vi "NanoValve Inject.vi"(8 "error in (no error)":errorcluster, 11 "VISA resource name":refnum<visa-resource-name>) -> (0 "error out":errorcluster)   [LabVIEW 2015]
uses:
  <vilib>/Instr/_visa.llb/VISA Configure Serial Port (Instr).vi
panel:
  out "return count":u32
  # "Inject Sample"
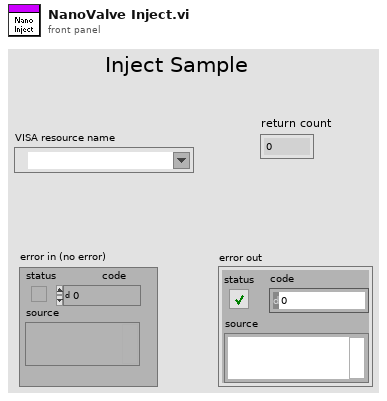
[diagram p1: front panel]
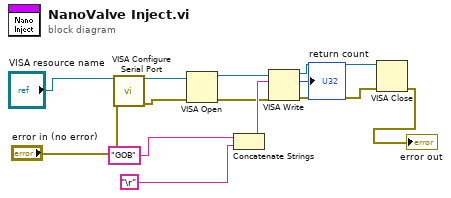
[diagram p0: block diagram]
diagram:
  n1 = call-poly "VISA Configure Serial Port"("VISA resource name"="VISA resource name", "error in (no error)"="error in (no error)") -> ("VISA resource name out"=w8:refnum<visa-resource-name>, "error out"=w7:errorcluster)  [unwired: 12 in]
  n2 = VISA Open(error in (no error)=w7, VISA resource name=w8) -> (VISA resource name=w10:refnum<visa-resource-name>, error out=w6:errorcluster)  [unwired: 3 in]
  n3 = Concatenate Strings("GOB", "\r") -> (w11:string)
  n4 = VISA Write(VISA resource name=w10, write buffer=w11, error in (no error)=w6) -> (VISA resource name out=w3:refnum<visa-resource-name>, return count=→"return count":u32, error out=w4:errorcluster)
  n5 = VISA Close(VISA resource name=w3, error in (no error)=w4) -> (error out=→"error out":errorcluster)
